vi "Server_Side.vi"() -> ()   [LabVIEW 2021]
panel:
  out "Channel":string
  out "LivingCurtians":u8(slide) scale=0.0..9.0
  out "LivingDoor":u8(slide) scale=0.0..2.0
  out "LivingLight":bool
  out "Volume":string
  out "tv on/off":bool
  out "BalconyLight3":bool
  out "BalconeLight1":bool
  out "BalconyLight2":bool
  out "KitchenCurtians":u8(slide) scale=0.0..9.0
  out "door 2":u8(slide) scale=0.0..2.0
  out "KitchenLight":bool
  out "MasterDoor":u8(slide) scale=0.0..2.0
  out "MasterCurtians":u8(slide) scale=0.0..9.0
  out "MasterLight1":bool
  out "MasterLight2":bool
  out "Bedroom2Door":u8(slide) scale=0.0..2.0
  out "Bedroom2Light":bool
  out "Bedroom1Door":u8(slide) scale=0.0..2.0
  out "Bedroom1Curtians":u8(slide) scale=0.0..9.0
  out "Bedroom2Curtians":u8(slide) scale=0.0..9.0
  out "Bedroom1Light":bool
  # "Kitchen"
  # "Bedroom - 2"
  # "Master Bedroom"
  # "Bedroom - 1"
  # "Volume:"
  # "Living Room"
  # "Channel:"
  # "Balcony"
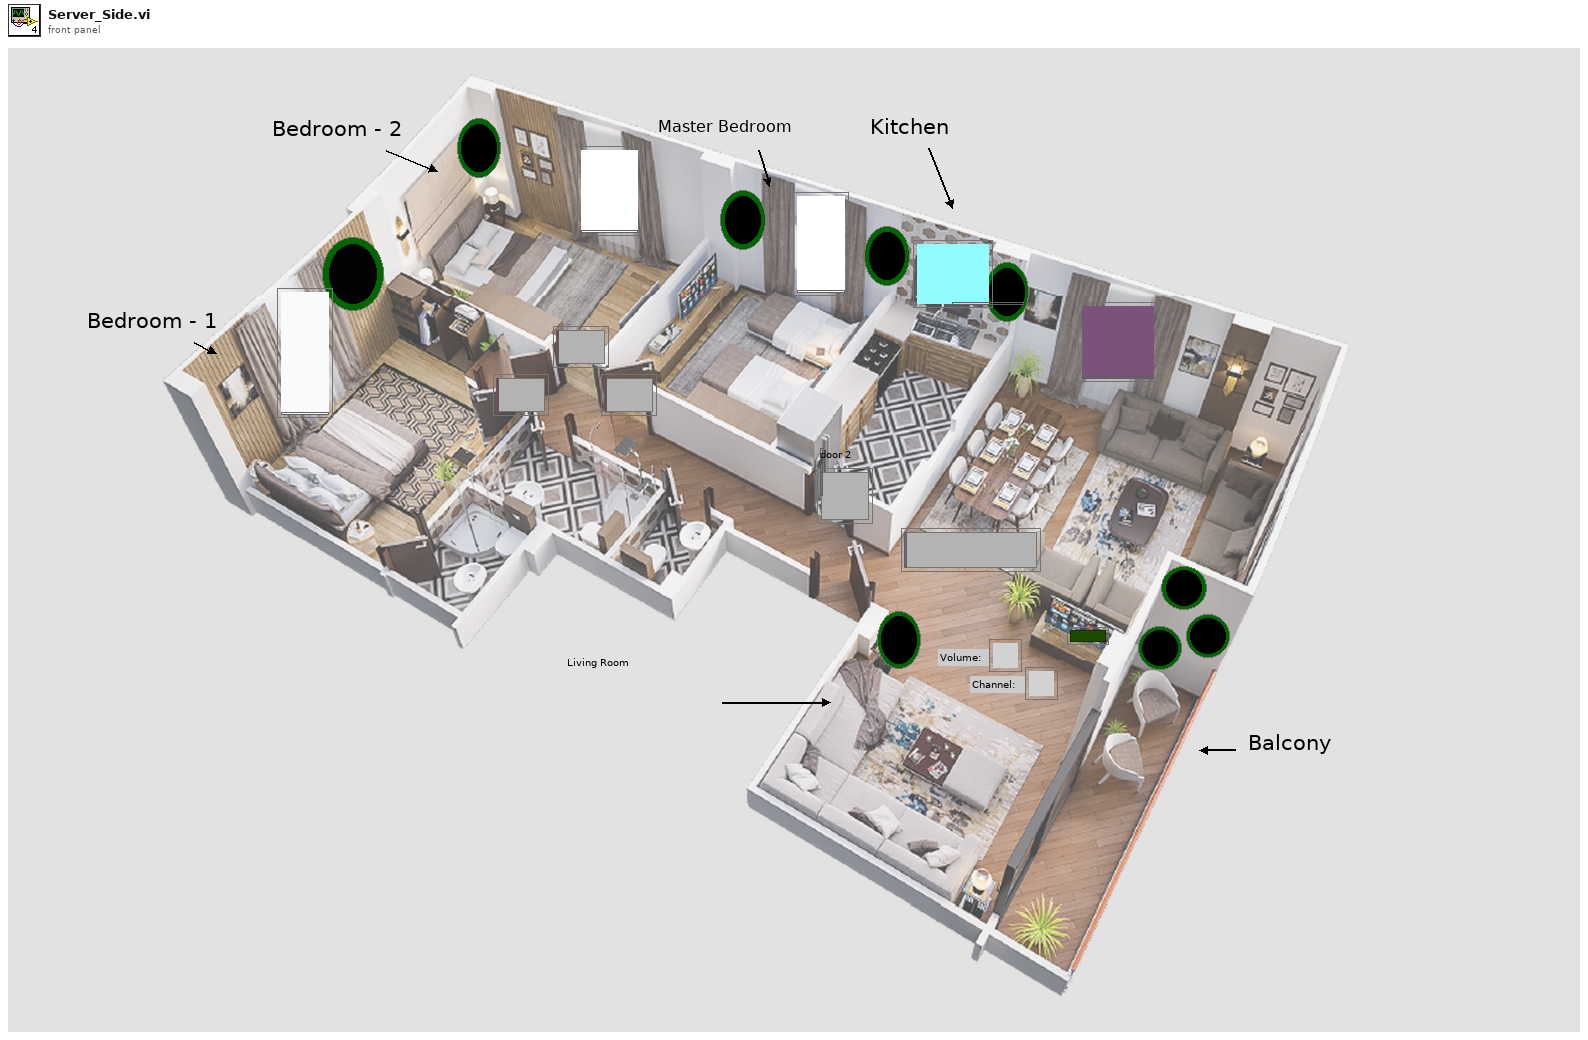
[diagram p1: front panel]
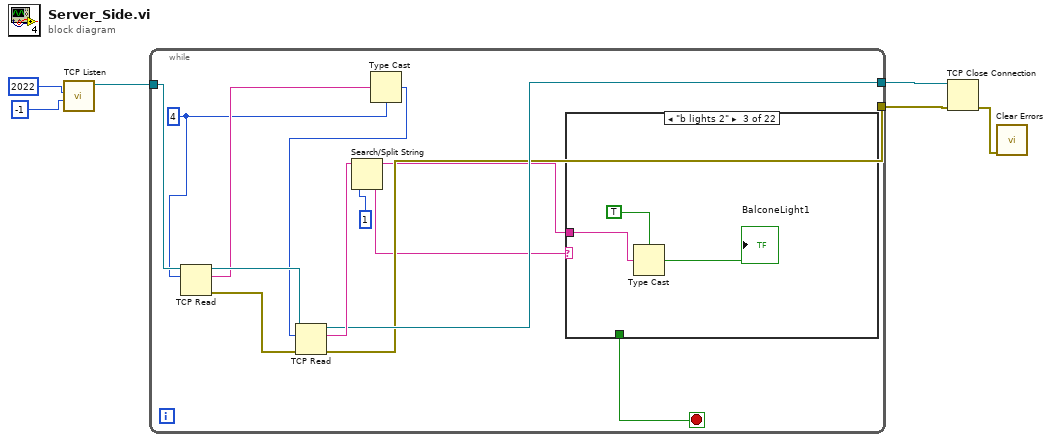
[diagram p0: block diagram]
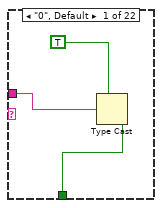
[diagram p2: hidden frame]
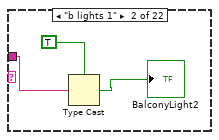
[diagram p3: hidden frame]
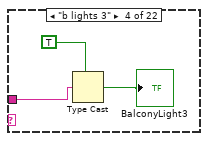
[diagram p4: hidden frame]
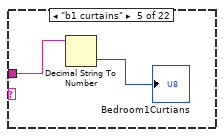
[diagram p5: hidden frame]
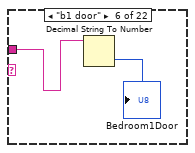
[diagram p6: hidden frame]
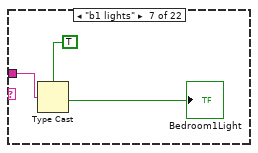
[diagram p7: hidden frame]
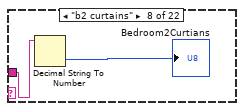
[diagram p8: hidden frame]
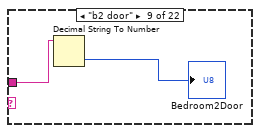
[diagram p9: hidden frame]
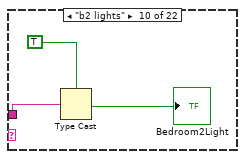
[diagram p10: hidden frame]
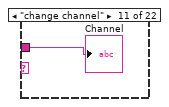
[diagram p11: hidden frame]
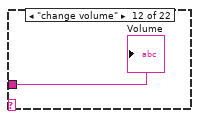
[diagram p12: hidden frame]
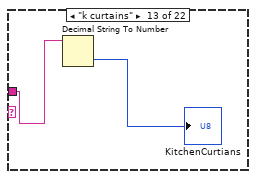
[diagram p13: hidden frame]
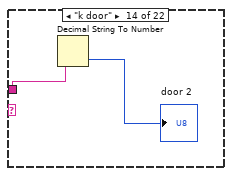
[diagram p14: hidden frame]
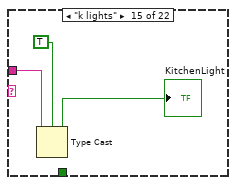
[diagram p15: hidden frame]
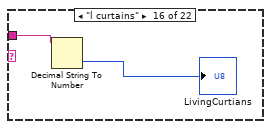
[diagram p16: hidden frame]
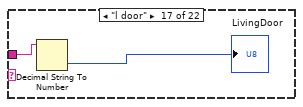
[diagram p17: hidden frame]
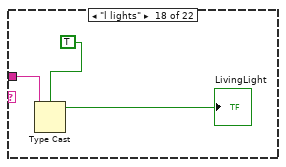
[diagram p18: hidden frame]
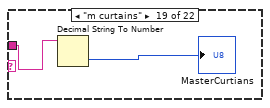
[diagram p19: hidden frame]
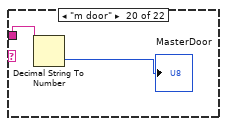
[diagram p20: hidden frame]
diagram:
  n1 = call <vilib>:"TCP Listen.vi"("timeout ms (wait forever: -1)"=-1, "port"=2022) -> ("connection ID"=w4:refnum<k5>)  [unwired: 5 in, 4 out]
  n2 = while {
    tunnel: w4 -> [w19]
    tunnel: [w13] -> w3
    tunnel: [w10] -> w2
    stop <- w12 stop-if-true
    w16 = 4
    n3 = TCP Read(connection ID=w19, bytes to read=w16) -> (connection ID out=w18:refnum<k5>, data out=w17:string, error out=w11:errorcluster)  [unwired: 3 in]
    n4 = Type Cast(type=w16, x=w17) -> (*(type *) &x=w9:i32)
    n5 = TCP Read(connection ID=w18, bytes to read=w9, error in (no error)=w11) -> (connection ID out=w13:refnum<k5>, data out=w15:string, error out=w10:errorcluster)  [unwired: 2 in]
    n6 = Search/Split String(string=w15, offset (0)=1) -> (substring before match=w7:string, match + rest of string=w8:string)  [unwired: 1 in, 1 out]
    n7 = case shown="\"b lights 2\"" w8 {
      tunnel: w7 -> [w22 w24 w26 w31 w33 w34 w37 w40 w41 w43 w46 w47 w48 w50 w52 w55 w57 w59 w62 w64 w67 w69]
      tunnel: [w20 _ _ _ _ _ _ _ _ _ _ _ _ _ _ _ _ _ _ _ _ _] -> w12
      frame "0", Default {
        n8 = Type Cast(type=TRUE, x=w22) -> (*(type *) &x=w20:bool)
      }
      frame "b lights 1" {
        n9 = Type Cast(type=TRUE, x=w24) -> (*(type *) &x=→"BalconyLight2":bool)
      }
      frame "b lights 2" {
        n10 = Type Cast(type=TRUE, x=w26) -> (*(type *) &x=→"BalconeLight1":bool)
      }
      frame "b lights 3" {
        n11 = Type Cast(type=TRUE, x=w31) -> (*(type *) &x=→"BalconyLight3":bool)
      }
      frame "b1 curtains" {
        n12 = Decimal String To Number(string=w33) -> (number=→"Bedroom1Curtians":i32)  [unwired: 2 in, 1 out]
      }
      frame "b1 door" {
        n13 = Decimal String To Number(string=w34) -> (number=→"Bedroom1Door":i32)  [unwired: 2 in, 1 out]
      }
      frame "b1 lights" {
        n14 = Type Cast(type=TRUE, x=w37) -> (*(type *) &x=→"Bedroom1Light":bool)
      }
      frame "b2 curtains" {
        n15 = Decimal String To Number(string=w40) -> (number=→"Bedroom2Curtians":i32)  [unwired: 2 in, 1 out]
      }
      frame "b2 door" {
        n16 = Decimal String To Number(string=w41) -> (number=→"Bedroom2Door":i32)  [unwired: 2 in, 1 out]
      }
      frame "b2 lights" {
        n17 = Type Cast(type=TRUE, x=w43) -> (*(type *) &x=→"Bedroom2Light":bool)
      }
      frame "change channel" {
        "Channel" <- w46
      }
      frame "change volume" {
        "Volume" <- w47
      }
      frame "k curtains" {
        n18 = Decimal String To Number(string=w48) -> (number=→"KitchenCurtians":i32)  [unwired: 2 in, 1 out]
      }
      frame "k door" {
        n19 = Decimal String To Number(string=w50) -> (number=→"door 2":i32)  [unwired: 2 in, 1 out]
      }
      frame "k lights" {
        n20 = Type Cast(type=TRUE, x=w52) -> (*(type *) &x=→"KitchenLight":bool)
      }
      frame "l curtains" {
        n21 = Decimal String To Number(string=w55) -> (number=→"LivingCurtians":i32)  [unwired: 2 in, 1 out]
      }
      frame "l door" {
        n22 = Decimal String To Number(string=w57) -> (number=→"LivingDoor":i32)  [unwired: 2 in, 1 out]
      }
      frame "l lights" {
        n23 = Type Cast(type=TRUE, x=w59) -> (*(type *) &x=→"LivingLight":bool)
      }
      frame "m curtains" {
        n24 = Decimal String To Number(string=w62) -> (number=→"MasterCurtians":i32)  [unwired: 2 in, 1 out]
      }
      frame "m door" {
        n25 = Decimal String To Number(string=w64) -> (number=→"MasterDoor":i32)  [unwired: 2 in, 1 out]
      }
      frame "m lights" {
        n26 = Type Cast(type=TRUE, x=w67) -> (*(type *) &x=→"MasterLight2" →"MasterLight1":bool)
      }
      frame "tv on/off" {
        n27 = Type Cast(type=TRUE, x=w69) -> (*(type *) &x=→"tv on/off":bool)
      }
    }
  }
  n28 = TCP Close Connection(connection ID=w3, error in (no error)=w2) -> (error out=w1:errorcluster)  [unwired: 1 in, 1 out]
  n29 = call <vilib>:"Clear Errors.vi"("error in (no error)"=w1) -> ()  [unwired: 5 in, 2 out]
